vi "AnalyzeRawData.vi"(8 "error in (no error)":errorcluster, 9 "Threshold, dB":dbl, 10 "Raw Data":waveform(dbl)[](array[waveform]), 11 "IIR Filter Specifications":T1) -> (0 "error out":errorcluster, 1 "Power Spectrum / PSD":cluster{"f0":dbl, "df":dbl, "magnitude":dbl[]}[](array[cluster]), 2 "Filtered Data":waveform(dbl)[](array[waveform]), 5 "Threshold Exceeded?":bool)   [LabVIEW 2019]
uses:
  <vilib>/measure/NI_MAPro.lvlib
  <vilib>/measure/maspectr.llb/FFT Power Spectrum and PSD for N Chan.vi
  <vilib>/measure/macond.llb/IIR Filter for N Chan.vi
  3f2c3bea-8526-4528-bf7d-44b8685116ad.vi
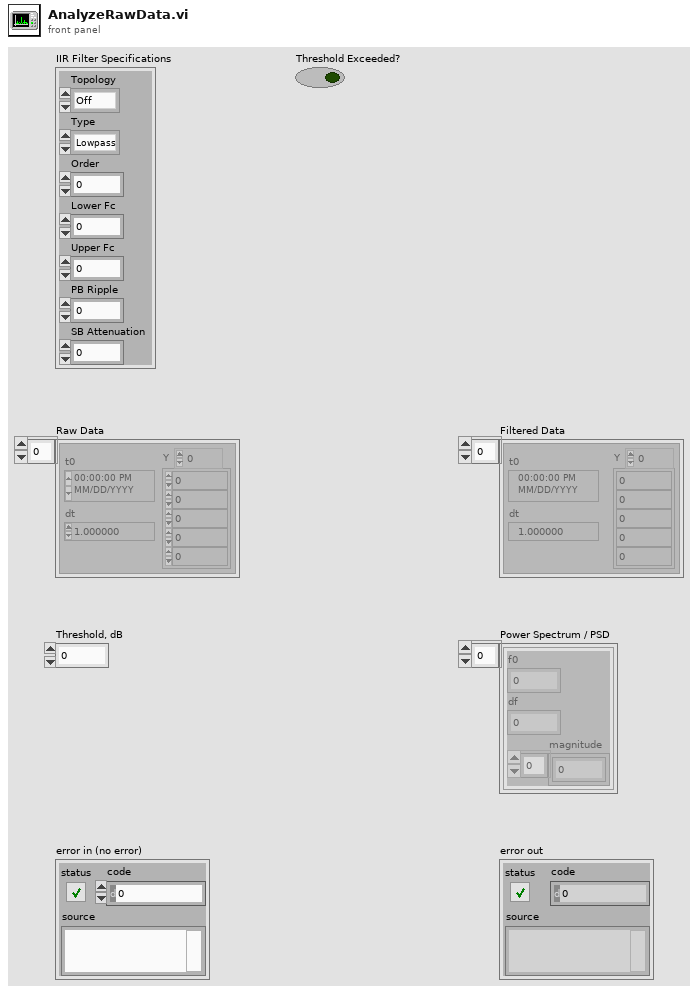
[diagram p1: front panel]
types:
  T1 = cluster{"Topology":enum16{"Off", "Butterworth", "Chebyshev", "Inverse Chebyshev", "Elliptic", "Bessel"}, "Type":enum16{"Lowpass", "Highpass", "Bandpass", "Bandstop"}, "Order":i32, "Lower Fc":dbl, "Upper Fc":dbl, "PB Ripple":dbl, "SB Attenuation":dbl}
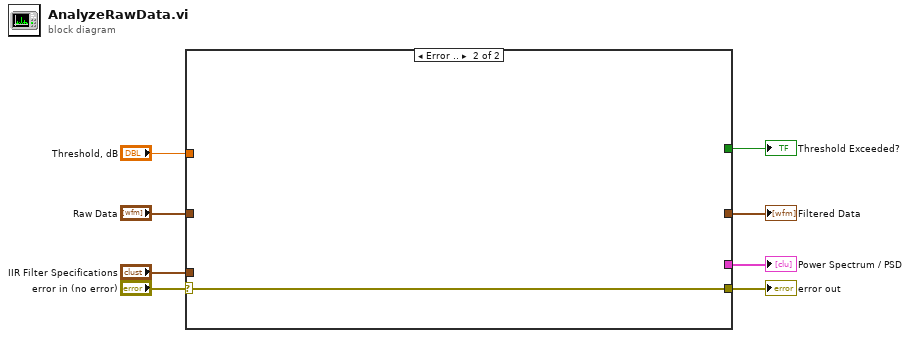
[diagram p0: block diagram]
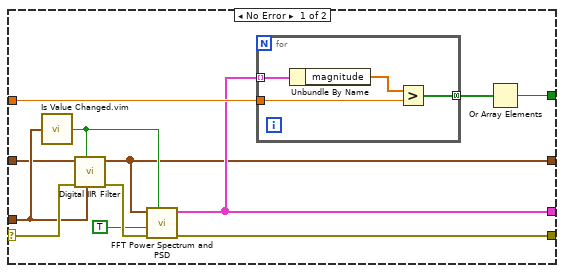
[diagram p2: hidden frame]
diagram:
  n1 = case shown="Error .." "error in (no error)" {
    selector: "error in (no error)" -> [w17 w25]
    tunnel: [w20 _] -> w8
    tunnel: [w19 w25] -> w7
    tunnel: "Threshold, dB" -> [w16 _]
    tunnel: [w15 _] -> w4
    tunnel: "IIR Filter Specifications" -> [w14 _]
    tunnel: [w12 _] -> w2
    tunnel: "Raw Data" -> [w11 _]
    frame No Error {
      n2 = call "Is Value Changed.vim"("value"=w14) -> ("changed or first call?"=w13:bool)
      n3 = call-poly <vilib>:"Digital IIR Filter.vi"("IIR filter specifications"=w14, "reset filters"=w13, "error in (no error)"=w17, "signal(s) in"=w11) -> ("error out"=w18:errorcluster, "signal(s) out"=w12:waveform(dbl)[])  [unwired: 5 in, 1 out]
      n4 = call-poly <vilib>:"FFT Power Spectrum and PSD.vi"("restart averaging (F)"=w13, "error in (no error)"=w18, "dB On (F)"=TRUE, "time signals"=w12) -> ("error out"=w19:errorcluster, "Power Spectrum / PSD"=w15:cluster{"f0":dbl, "df":dbl, "magnitude":dbl[]}[])  [unwired: 4 in, 2 out]
      n5 = for {
        tunnel: [w23] -> w10 mode=concatenating
        tunnel: w15 -> [w22] mode=indexing
        tunnel: w16 -> [w21]
        n6 = Unbundle By Name(w22) -> ("magnitude"=w24:dbl[])
        n7 = Greater?(x=w24, y=w21) -> (0:w23:bool[])
      }
      n8 = Or Array Elements(Boolean array=w10) -> (logical OR=w20:bool)
    }
    frame Error {
    }
  }
  "Threshold Exceeded?" <- w8
  "error out" <- w7
  "Power Spectrum / PSD" <- w4
  "Filtered Data" <- w2
